vi "black box state code.vi"(10 "value in":dbl, 11 "state in":u8) -> (2 "value out":dbl, 3 "state out":u8)   [LabVIEW 2013, in "user tag bus module.lvclass"]
uses:
  user tag bus module.lvclass
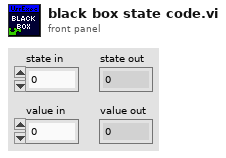
[diagram p1: front panel]
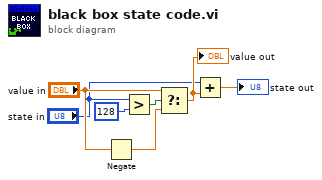
[diagram p0: block diagram]
diagram:
  n1 = Negate(x="value in") -> (-x=w5:dbl)
  n2 = Greater?(x="state in", y=u8 128) -> (0:w4:bool)
  n3 = Select(t="value in", s=w4, f=w5) -> (s? t:f=w7:dbl)
  "value out" <- w7
  n4 = Add(x="state in", y=w7) -> (x+y=→"state out":dbl)
